vi "Control loop new type.vi"(8 "error in":errorcluster) -> (0 "error out":errorcluster)   [LabVIEW 2011]
uses:
  Control loop state.ctl
  Robot Global Data.vi
  <vilib>/addons/control/pid/pid.llb/PID (DBL).vi
  <vilib>/addons/control/pid/NI_PID_pid.lvlib
panel:
  in  "Tolerance (degrees)":dbl
  out "State":T1
  in  "Turret Span / 2":dbl
  in  "Gyro Lock PID gains":T2={"proportional gain (Kc)"=1.0, "integral time (Ti, min)"=0.01, "derivative time (Td, min)"=0.0} {"derivative time (Td, min)" format="%.3f"; "integral time (Ti, min)" format="%.3f"; "proportional gain (Kc)" format="%.3f"}
  in  "Lock On PID gains":T2={"proportional gain (Kc)"=1.0, "integral time (Ti, min)"=0.01, "derivative time (Td, min)"=0.0} {"derivative time (Td, min)" format="%.3f"; "integral time (Ti, min)" format="%.3f"; "proportional gain (Kc)" format="%.3f"}
  in  "Basket forward offset":dbl
  out "Error":dbl
  in  "Pixel tolerance":dbl
  in  "Still Tracking PID gains":T2={"proportional gain (Kc)"=1.0, "integral time (Ti, min)"=0.01, "derivative time (Td, min)"=0.0} {"derivative time (Td, min)" format="%.3f"; "integral time (Ti, min)" format="%.3f"; "proportional gain (Kc)" format="%.3f"}
  in  "Idle Tracking PID gains":T2={"proportional gain (Kc)"=1.0, "integral time (Ti, min)"=0.01, "derivative time (Td, min)"=0.0} {"derivative time (Td, min)" format="%.3f"; "integral time (Ti, min)" format="%.3f"; "proportional gain (Kc)" format="%.3f"}
  # "Constants--do not change!\nBehavior of changing these constants is\ndeliberately undefined by any specification."
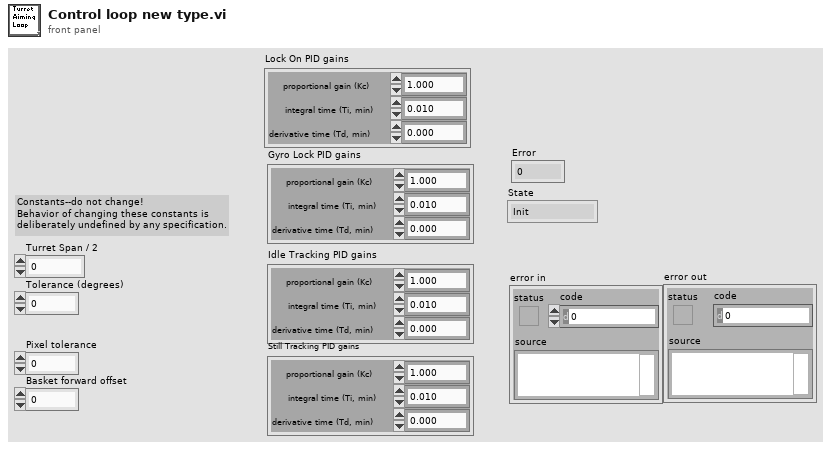
[diagram p1: front panel]
types:
  T1 = typedef "Control loop state.ctl" = enum16{"Init", "Track", "Calculate", "Lock On", "Idle", "Gyro Lock", "Out of Bounds"}
  T2 = cluster{"proportional gain (Kc)":dbl, "integral time (Ti, min)":dbl, "derivative time (Td, min)":dbl}
  T3 = typedef "BasketType.ctl" = enum16{"Left", "Bottom", "Right", "Top"}
  T4 = typedef "WPI_MotorControlDeviceRef.ctl" = cluster{"DeviceStatus":errorcluster, "Type":enum16{"PWM", "CAN"}, "PWM":cluster{"Digital Module":T5, "PWM Channel":T6, "DeadBand":T7}, "CAN":cluster{"Device Number":u8, "Control Mode":T8, "Semaphore":T9, "Max Vout":dbl}, "Invert":bool, "TransformRef":T10, "InvTransformRef":T10}
  T5 = typedef "FPGA_TypedefDigitalModule.ctl" = enum16{"Digital Module 1", "Digital Module 2"}
  T6 = typedef "FPGA_DIOPWMChannel.ctl" = enum8{"PWM 1", "PWM 2", "PWM 3", "PWM 4", "PWM 5", "PWM 6", "PWM 7", "PWM 8", "PWM 9", "PWM 10", "Invalid"}
  T7 = typedef "WPI_PWMDeadband.ctl" = cluster{"Name":string, "maxPositivePwm":i32, "minPositivePwm":i32, "centerPwm":i32, "maxNegativePwm":i32, "minNegativePwm":i32, "angularRange":u16}
  T8 = typedef "WPI_CANJaguar_ControlMode.ctl" = enum8{"Percent VBus", "Current", "Speed", "Position", "Voltage"}
  T9 = typedef "Semaphore RefNum" = refnum<k1>
  T10 = typedef "WPI_PWMTransform_ConPane.ctl" = refnum<vi>
  T11 = typedef "WPI_GyroDevRef.ctl" = cluster{"DevStatus":errorcluster, "Analog Module":T12, "Analog Channel":T13, "Offset":dbl, "Gain (VoltsPerDegree/Second)":dbl}
  T12 = typedef "FPGA_TypedefAnalogModule.ctl" = enum16{"Analog Module 1", "Analog Module 2"}
  T13 = typedef "FPGA_AIChannel.ctl" = enum8{"AI 1", "AI 2", "AI 3", "AI 4", "AI 5", "AI 6", "AI 7", "AI 8", "Invalid"}
  T14 = typedef "TurretDevRef.ctl" = cluster{"MotorControlDevRef":T4, "LauncherGyro":T11, "RobotGyro":T11, "Difference Range":cluster{"Max Difference":dbl, "Min Difference":dbl}, "Dead Band Tolerance":dbl}
  T15 = cluster{"Position":cluster{"X":dbl, "Y":dbl}, "Distance (ft)":dbl, "Target Corners":cluster{"Bottom Left":cluster{"X":dbl, "Y":dbl}, "Bottom Right":cluster{"X":dbl, "Y":dbl}, "Top Right":cluster{"X":dbl, "Y":dbl}, "Top Left":cluster{"X":dbl, "Y":dbl}}}[]
  T16 = cluster{"Position":cluster{"X":dbl, "Y":dbl}, "Distance (ft)":dbl, "Target Corners":cluster{"Bottom Left":cluster{"X":dbl, "Y":dbl}, "Bottom Right":cluster{"X":dbl, "Y":dbl}, "Top Right":cluster{"X":dbl, "Y":dbl}, "Top Left":cluster{"X":dbl, "Y":dbl}}}
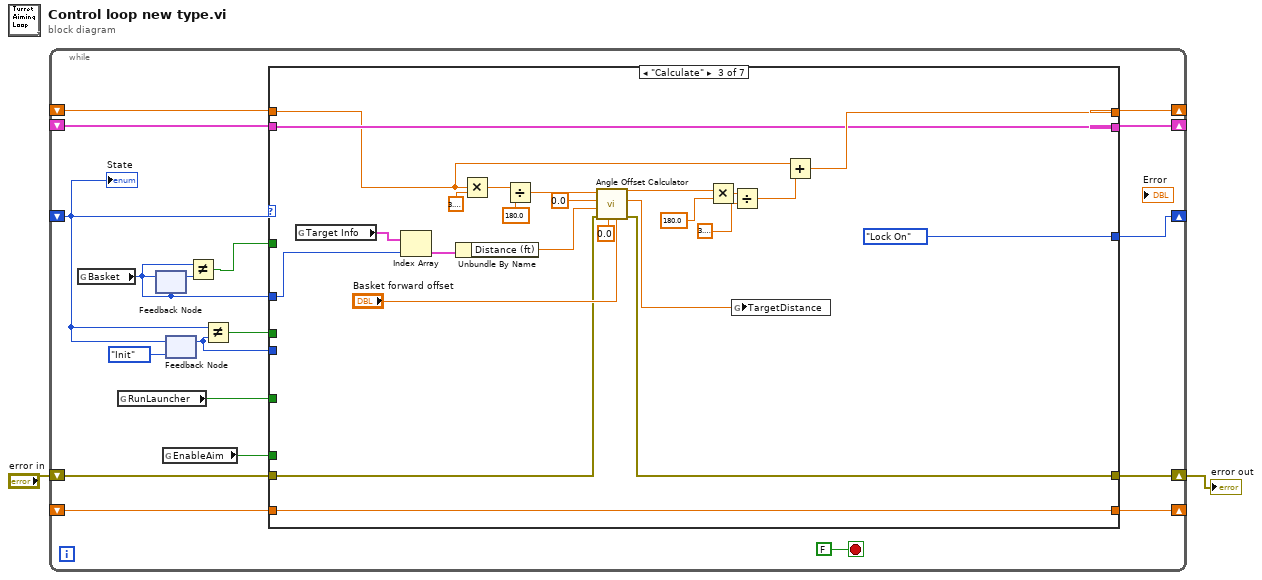
[diagram p0: block diagram]
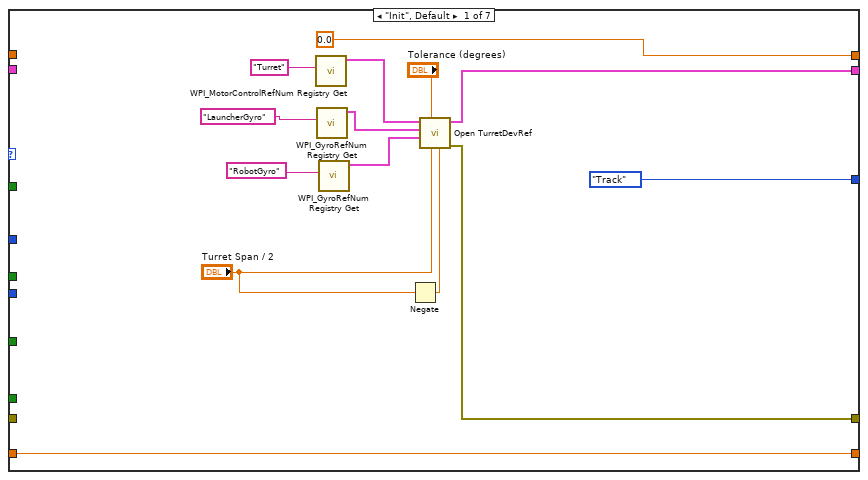
[diagram p2: hidden frame]
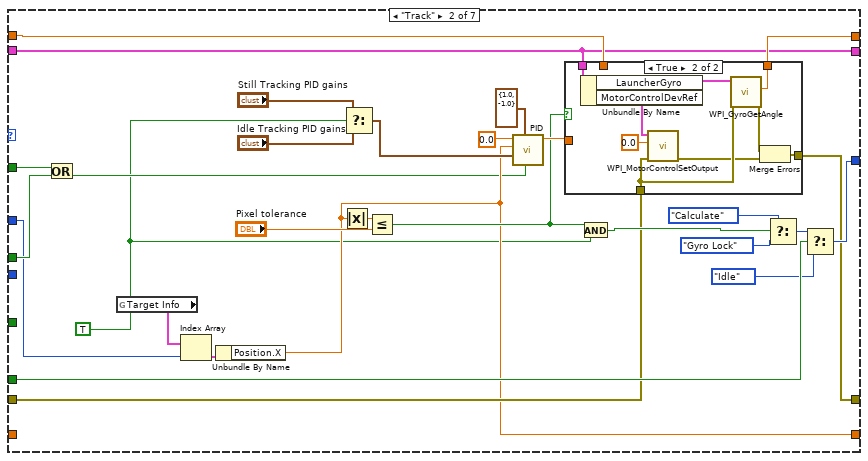
[diagram p3: hidden frame]
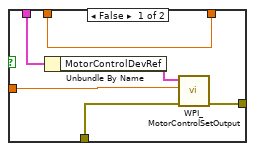
[diagram p4: hidden frame]
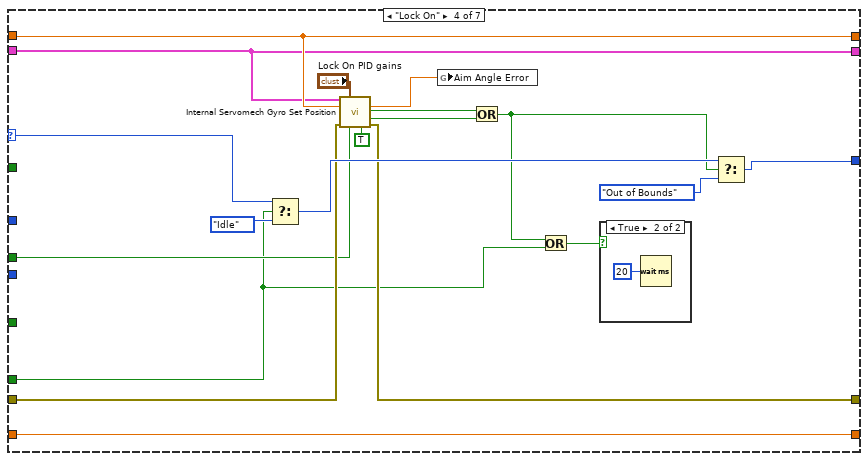
[diagram p5: hidden frame]
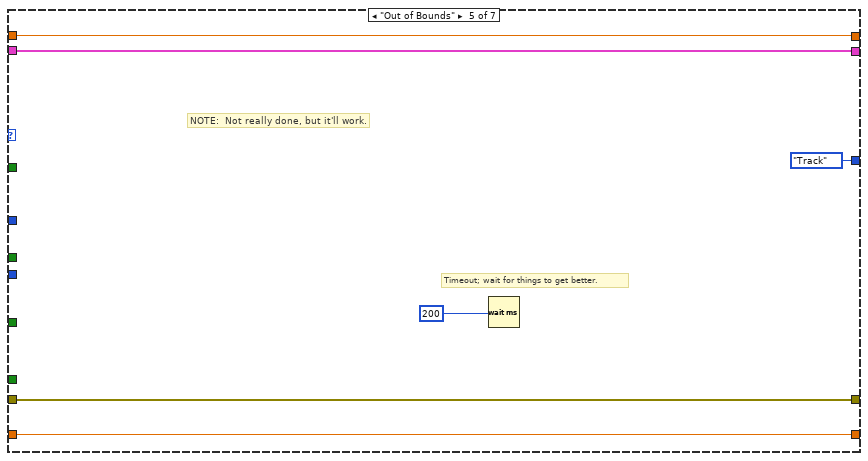
[diagram p7: hidden frame]
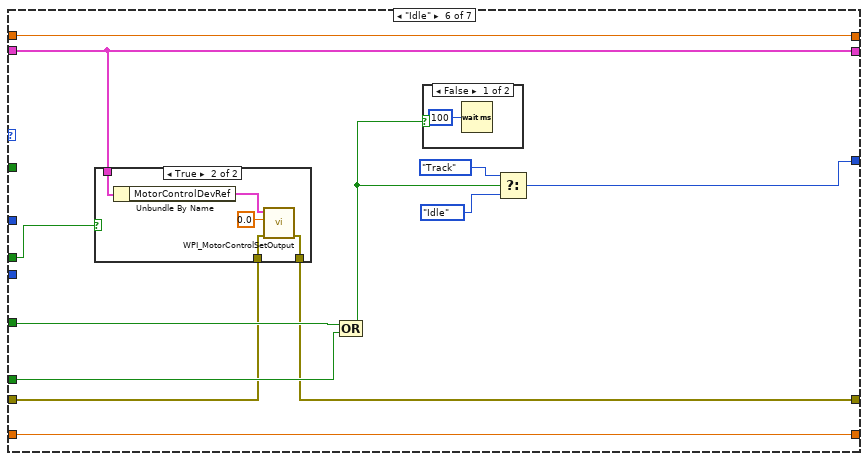
[diagram p8: hidden frame]
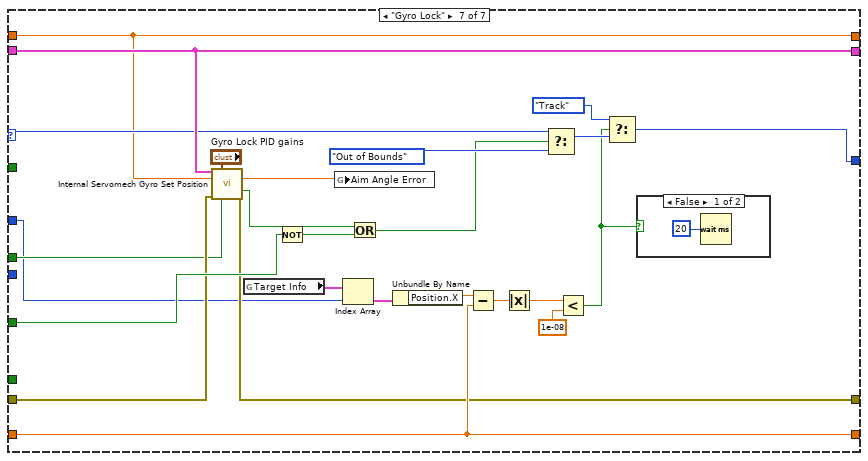
[diagram p11: hidden frame]
diagram:
  n1 = while {
    shift-right: [w21] -> _
    shift-left: _ -> [w20]
    shift-right: [w18] -> _
    shift-left: _ -> [w6]
    shift-right: [w17] -> _
    shift-left: _ -> [w16]
    shift-right: [w13] -> _
    shift-left: _ -> [w12]
    shift-right: [w9] -> w1
    shift-left: "error in" -> [w10]
    stop <- FALSE stop-if-true
    n2 = global read "Robot Global Data.vi" "Basket"() -> (w3:T3)
    n3 = global read "Robot Global Data.vi" "RunLauncher"() -> (w8:bool)
    n4 = feedback #1(w3) -> (w7:T3)
    n5 = feedback-in #1(w3) -> ()
    n6 = global read "Robot Global Data.vi" "EnableAim"() -> (w14:bool)
    n7 = feedback-in #2(w6) -> ()
    n8 = feedback #2(Control_loop_state."Init" ("Mode 2")) -> (w15:T1)
    n9 = Not Equal?(x=w3, y=w7) -> (x != y?=w4:bool)
    n10 = Not Equal?(x=w6, y=w15) -> (x != y?=w5:bool)
    n11 = case shown="\"Calculate\"" w6 {
      selector: w6 -> [_ _ _ w118 _ _ w168]
      tunnel: [0.0 w57 w95 w116 w129 w137 w167] -> w21
      tunnel: w20 -> [_ w56 w89 w116 w129 w137 w167]
      tunnel: w5 -> [_ w52 _ w111 _ w134 w154]
      tunnel: [Control_loop_state."Track" ("Mode 2") w45 Control_loop_state."Lock On" ("Mode 2") w121 Control_loop_state."Track" ("Mode 2") w130 w170] -> w18
      tunnel: w8 -> [_ _ _ _ _ w139 w164]
      tunnel: [w27 w55 w93 w110 w128 w133 w169] -> w17
      tunnel: w16 -> [_ w55 w93 w110 w128 w133 w169]
      tunnel: w15 -> [_ _ _ _ _ _ _]
      tunnel: w14 -> [_ w47 _ w106 _ w136 _]
      tunnel: [w24 w40 w88 w114 w125 w135 w160] -> w13
      tunnel: w12 -> [w24 _ w88 w114 w125 w135 w160]
      tunnel: w10 -> [_ w44 w87 w113 w124 w132 w156]
      tunnel: [w23 w43 w86 w112 w124 w131 w155] -> w9
      tunnel: w4 -> [_ w38 _ _ _ _ _]
      tunnel: w3 -> [_ w37 w80 _ _ _ w152]
      frame "Init", Default {
        n12 = call <vilib>:"WPI_MotorControlRefNum Registry Get.vi"("refnum name"="Turret") -> ("MotorControlDevRef"=w31:T4)  [unwired: 9 in, 1 out]
        n13 = call <vilib>:"WPI_GyroRefNum Registry Get.vi"("refnum name"="LauncherGyro") -> ("GyroDevRef"=w30:T11)  [unwired: 9 in, 1 out]
        n14 = call <vilib>:"WPI_GyroRefNum Registry Get.vi"("refnum name"="RobotGyro") -> ("GyroDevRef"=w28:T11)  [unwired: 9 in, 1 out]
        n15 = Negate(x="Turret Span / 2") -> (-x=w25:dbl)
        n16 = call "Open TurretDevRef.vi"("Min Difference"=w25, "Max Difference"="Turret Span / 2", "Dead Band Tolerance"="Tolerance (degrees)", "RobotGyro"=w28, "LauncherGyro"=w30, "MotorControlDevRef"=w31) -> ("error out"=w23:errorcluster, "TurretDevRef"=w27:T14)  [unwired: 4 in]
      }
      frame "Track" {
        w36 = TRUE
        n17 = Or(x=w38, y=w52) -> (x .or. y?=w39:bool)
        n18 = global read "Robot Global Data.vi" "Target Info"() -> (w42:T15)
        n19 = Index Array(array=w42, index=w37) -> (element=w41:T16)
        n20 = Unbundle By Name(w41) -> ("Position.X"=w40:dbl)
        n21 = Absolute Value(x=w40) -> (abs(x)=w60:dbl)
        n22 = Select(t="Still Tracking PID gains", s=w36, f="Idle Tracking PID gains") -> (s? t:f=w61:T2)
        n23 = Less Or Equal?(x=w60, y="Pixel tolerance") -> (x <= y?=w53:bool)
        n24 = call-poly <vilib>:"PID.vi"("reinitialize? (F)"=w39, "output range"=cluster{"output high":dbl, "output low":dbl} {"output high"=1.0, "output low"=-1.0}, "PID gains"=w61, "process variable"=w40, "setpoint"=0.0) -> ("output"=w54:dbl)  [unwired: 5 in, 1 out]
        n25 = case shown="True" w53 {
          tunnel: [w70 w79] -> w57
          tunnel: w56 -> [w70 _]
          tunnel: w54 -> [w69 _]
          tunnel: w55 -> [w68 w78]
          tunnel: w44 -> [w66 w75]
          tunnel: [w65 w71] -> w43
          frame False {
            n26 = Unbundle By Name(w68) -> ("MotorControlDevRef"=w67:T4)
            n27 = call <vilib>:"WPI_MotorControlSetOutput.vi"("error in (no error)"=w66, "Output"=w69, "MotorControlDevRef"=w67) -> ("error out"=w65:errorcluster)  [unwired: 7 in, 1 out]
          }
          frame True {
            n28 = Unbundle By Name(w78) -> ("LauncherGyro"=w77:T11, "MotorControlDevRef"=w76:T4)
            n29 = call <vilib>:"WPI_MotorControlSetOutput.vi"("error in (no error)"=w75, "Output"=0.0, "MotorControlDevRef"=w76) -> ("error out"=w72:errorcluster)  [unwired: 7 in, 1 out]
            n30 = call <vilib>:"WPI_GyroGetAngle.vi"("error in (no error)"=w75, "GyroDevRef"=w77) -> ("error out"=w73:errorcluster, "Angle"=w79:dbl)  [unwired: 6 in, 2 out]
            n31 = Merge Errors(w73, w72) -> (w71:errorcluster)
          }
        }
        n32 = And(x=w53, y=w36) -> (x .and. y?=w51:bool)
        n33 = Select(t=Control_loop_state."Calculate" ("Mode 2"), s=w51, f=Control_loop_state."Gyro Lock" ("Mode 2")) -> (s? t:f=w48:T1)
        n34 = Select(t=w48, s=w47, f=Control_loop_state."Idle") -> (s? t:f=w45:T1)
      }
      frame "Calculate" {
        n35 = global read "Robot Global Data.vi" "Target Info"() -> (w83:T15)
        n36 = Index Array(array=w83, index=w80) -> (element=w82:T16)
        n37 = Unbundle By Name(w82) -> ("Distance (ft)"=w81:dbl)
        n38 = Multiply(x=w89, y=3.141592653589793) -> (x*y=w97:dbl)
        n39 = Divide(x=w97, y=180.0) -> (x/y=w101:dbl)
        n40 = call "Angle Offset Calculator.vi"("Basket forward offset"="Basket forward offset", "Camera forward of turret"=0.0, "error in (no error)"=w87, "Target Distance"=w81, "Basket X offset"=0.0, "Turret Gyro (Radians)"=w101) -> ("error out"=w86:errorcluster, "Distance"=w84:dbl, "Angle Offset"=w102:dbl)  [unwired: 3 in]
        n41 = Multiply(x=w102, y=180.0) -> (x*y=w98:dbl)
        n42 = Divide(x=w98, y=3.141592653589793) -> (x/y=w90:dbl)
        n43 = global write "Robot Global Data.vi" "TargetDistance"(w84) -> ()
        n44 = Add(x=w89, y=w90) -> (x+y=w95:dbl)
      }
      frame "Lock On" {
        n45 = Select(t=w118, s=w106, f=Control_loop_state."Idle" ("Mode 2")) -> (s? t:f=w120:T1)
        n46 = call "Internal Servomech Gyro Set Position.vi"("TurretDevRef"=w110, "PID gains"="Lock On PID gains", "Desired Gyro position"=w116, "error in"=w113, "reinitialize? (F)"=w111, "Use dead band?"=TRUE) -> ("Error"=w107:dbl, "Hit dead band?"=w108:bool, "In Range?"=w115:bool, "error out"=w112:errorcluster)  [unwired: 5 in, 1 out]
        n47 = global write "Robot Global Data.vi" "Aim Angle Error"(w107) -> ()
        n48 = Or(x=w108, y=w115) -> (x .or. y?=w105:bool)
        n49 = Or(x=w105, y=w106) -> (x .or. y?=w104:bool)
        n50 = case shown="True" w104 {
          frame False {
          }
          frame True {
            n51 = Wait (ms)(milliseconds to wait=u32 20) -> ()  [unwired: 1 out]
          }
        }
        n52 = Select(t=w120, s=w105, f=Control_loop_state."Out of Bounds" ("Mode 2")) -> (s? t:f=w121:T1)
      }
      frame "Out of Bounds" {
        # "Timeout; wait for things to get better."
        # "NOTE:  Not really done, but it'll work."
        n53 = Wait (ms)(milliseconds to wait=200) -> ()  [unwired: 1 out]
      }
      frame "Idle" {
        n54 = case shown="True" w134 {
          tunnel: w133 -> [_ w146]
          tunnel: w132 -> [w142 w144]
          tunnel: [w142 w143] -> w131
          frame False {
          }
          frame True {
            n55 = Unbundle By Name(w146) -> ("MotorControlDevRef"=w145:T4)
            n56 = call <vilib>:"WPI_MotorControlSetOutput.vi"("error in (no error)"=w144, "Output"=0.0, "MotorControlDevRef"=w145) -> ("error out"=w143:errorcluster)  [unwired: 7 in, 1 out]
          }
        }
        n57 = Compound Arithmetic op=OR(w139, w136) -> (w138:bool)
        n58 = case shown="False" w138 {
          frame False {
            n59 = Wait (ms)(milliseconds to wait=u32 100) -> ()  [unwired: 1 out]
          }
          frame True {
          }
        }
        n60 = Select(t=Control_loop_state."Track" ("Mode 2"), s=w138, f=Control_loop_state."Idle" ("Mode 2")) -> (s? t:f=w130:T1)
      }
      frame "Gyro Lock" {
        n61 = call "Internal Servomech Gyro Set Position.vi"("TurretDevRef"=w169, "PID gains"="Gyro Lock PID gains", "Desired Gyro position"=w167, "error in"=w156, "reinitialize? (F)"=w154) -> ("Error"=w149:dbl, "In Range?"=w163:bool, "error out"=w155:errorcluster)  [unwired: 6 in, 2 out]
        n62 = global read "Robot Global Data.vi" "Target Info"() -> (w153:T15)
        n63 = Not(x=w164) -> (.not. x?=w165:bool)
        n64 = global write "Robot Global Data.vi" "Aim Angle Error"(w149) -> ()
        n65 = Index Array(array=w153, index=w152) -> (element=w151:T16)
        n66 = Or(x=w163, y=w165) -> (x .or. y?=w162:bool)
        n67 = Unbundle By Name(w151) -> ("Position.X"=w150:dbl)
        n68 = Subtract(x=w150, y=w160) -> (x-y=w161:dbl)
        n69 = Absolute Value(x=w161) -> (abs(x)=w159:dbl)
        n70 = Select(t=w168, s=w162, f=Control_loop_state."Out of Bounds" ("Mode 2")) -> (s? t:f=w172:T1)
        n71 = Less?(x=w159, y=1e-08) -> (x < y?=w157:bool)
        n72 = Select(t=Control_loop_state."Track" ("Mode 2"), s=w157, f=w172) -> (s? t:f=w170:T1)
        n73 = case shown="False" w157 {
          frame False {
            n74 = Wait (ms)(milliseconds to wait=u32 20) -> ()  [unwired: 1 out]
          }
          frame True {
          }
        }
      }
    }
    "State" <- w6
  }
  "error out" <- w1
